vi "CreateHTML.vi"(0 "reference in":refnum<class "Text.lvclass">, 2 "VI Name":string, 5 "error in (no error)":errorcluster) -> (13 "script dependencies":string[](array[string]), 14 "reference out":refnum<class "Text.lvclass">, 15 "HTML":string, 16 "js variables":string, 17 "js code for controls":string, 18 "js code for indicators":string, 19 "error out":errorcluster)   [LabVIEW 2014, in "FrontPanelPublisher.lvlib" / "Text.lvclass"]
uses:
  Text.lvclass
  Object_class/Object.lvclass
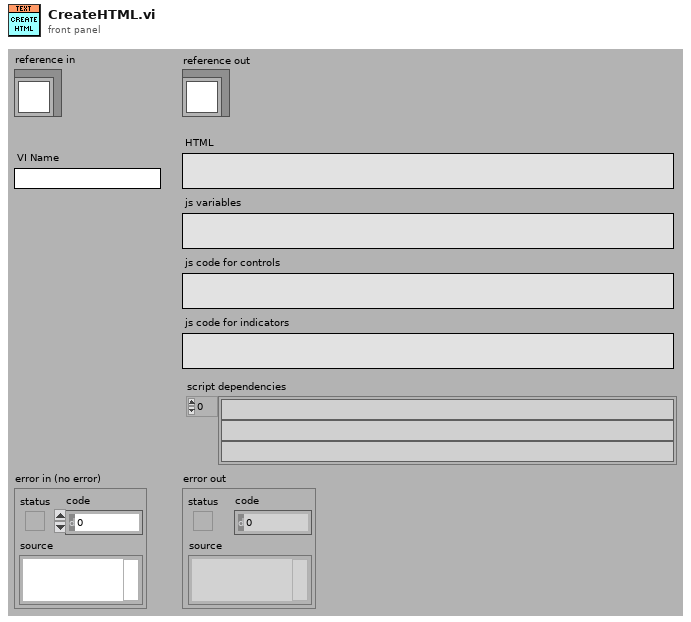
[diagram p1: front panel]
types:
  T1 = typedef "FrontPanelPublisher.lvlib/Object.lvclass/Attributes.ctl" = cluster{"UID":i32, "Type":string, "Coordinates":T2, "Reference":refnum<vi>}
  T2 = typedef "FrontPanelPublisher.lvlib/Object.lvclass/Coordinates.ctl" = cluster{"Left":i32, "Top":i32, "Height":u32, "Width":u32}
  T3 = typedef "FrontPanelPublisher.lvlib/Text.lvclass/Attributes.ctl" = cluster{"Text":string, "Font":string, "Font Size":u32, "Visible":bool}
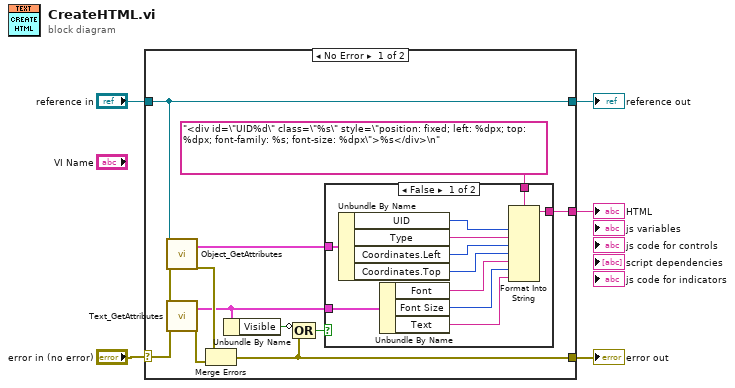
[diagram p0: block diagram]
diagram:
  n1 = case shown="No Error" "error in (no error)" {
    selector: "error in (no error)" -> [w15 w29]
    tunnel: [w13 w29] -> w4
    tunnel: [w9 w28] -> w2
    tunnel: "reference in" -> [w9 w28]
    tunnel: [w10 _] -> w1
    frame No Error {
      n2 = call "Object_GetAttributes.vi"("reference in"=w9, "error in (no error)"=w15) -> ("Data"=w11:T1, "error out"=w14:errorcluster)  [unwired: 14 in, 2 out]
      n3 = call "Text_GetAttributes.vi"("reference in"=w9) -> ("Data"=w8:T3, "error out"=w16:errorcluster)  [unwired: 15 in, 2 out]
      n4 = Merge Errors(w14, w16) -> (w13:errorcluster)
      n5 = Unbundle By Name(w8) -> ("Visible"=w7:bool)
      n6 = Compound Arithmetic op=OR(invert w7, w13) -> (w6:bool)
      n7 = case shown="False" w6 {
        tunnel: "<div id=\"UID%d\" class=\"%s\" style=\"position: fixed; left: %dpx; top: %dpx; font-family: %s; font-size: %dpx\">%s</div>\n" -> [w27 _]
        tunnel: w11 -> [w26 _]
        tunnel: [w21 _] -> w10
        tunnel: w8 -> [w20 _]
        frame False {
          n8 = Unbundle By Name(w26) -> ("UID"=w25:i32, "Type"=w24:string, "Coordinates.Left"=w23:i32, "Coordinates.Top"=w22:i32)
          n9 = Unbundle By Name(w20) -> ("Font"=w18:string, "Font Size"=w17:u32, "Text"=w19:string)
          n10 = Format Into String(format string=w27, w25, w24, w23, w22, w18, w17, w19) -> (resulting string=w21:string)  [unwired: 2 in, 1 out]
        }
        frame True {
        }
      }
    }
    frame Error {
    }
  }
  "error out" <- w4
  "reference out" <- w2
  "HTML" <- w1
